vi "Untitled 1.vi"() -> ()   [LabVIEW 2017]
uses:
  UI Error Handlers/support/Message Queue/Message Cluster.ctl
  UI Error Handlers/support/Message Queue/Message Queue.lvlib
panel:
  out "error out":errorcluster
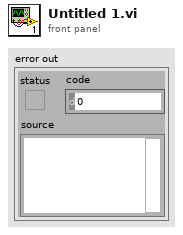
[diagram p1: front panel]
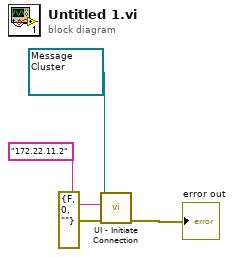
[diagram p0: block diagram]
diagram:
  n1 = call "UI - Initiate Connection.vi"("error in (no error)"=errorcluster {"status"=FALSE, "code"=0, "source"=""}, "Controller Address"="172.22.11.2", "Message Queue"=refnum<queue> refnum) -> ("error out"=→"error out":errorcluster)  [unwired: 7 in, 1 out]
